vi "FGV_REWORK_login.vi"(6 "login_refnums":T1, 7 "options":T2, 8 "error_in":errorcluster, 9 "access_level_in":i32, 10 "username_in":string, 11 "ID_in":string) -> (0 "error_out":errorcluster, 1 "access_level_out":i32, 2 "username_out":string, 3 "ID_out":string)   [LabVIEW 2019]
uses:
  FGV_REWORK_login.ctl
  REWORK_login_refnums.ctl
  REWORK_destination_selector/FGV_REWORK_destination_selector.ctl
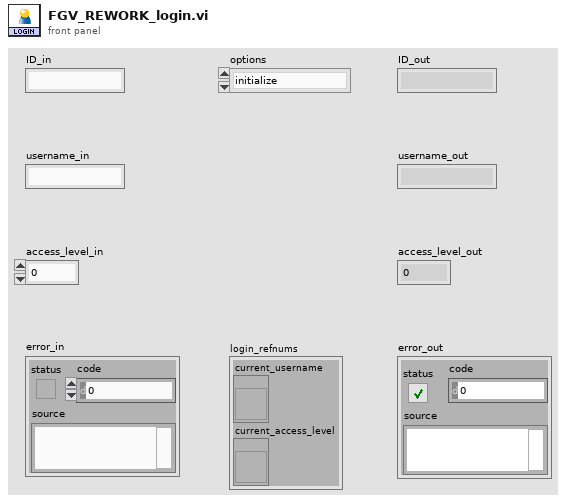
[diagram p1: front panel]
types:
  T1 = typedef "REWORK_login_refnums.ctl" = cluster{"current_username":refnum<vi>, "current_access_level":refnum<vi>}
  T2 = typedef "FGV_REWORK_login.ctl" = enum16{"initialize", "login", "logout", "get_login_info"}
  T3 = typedef "FGV_REWORK_destination_selector.ctl" = enum16{"initialize", "set_values", "display_values", "set_new_login", "enable", "disable", "disable_gray", "get_rework_to", "clear"}
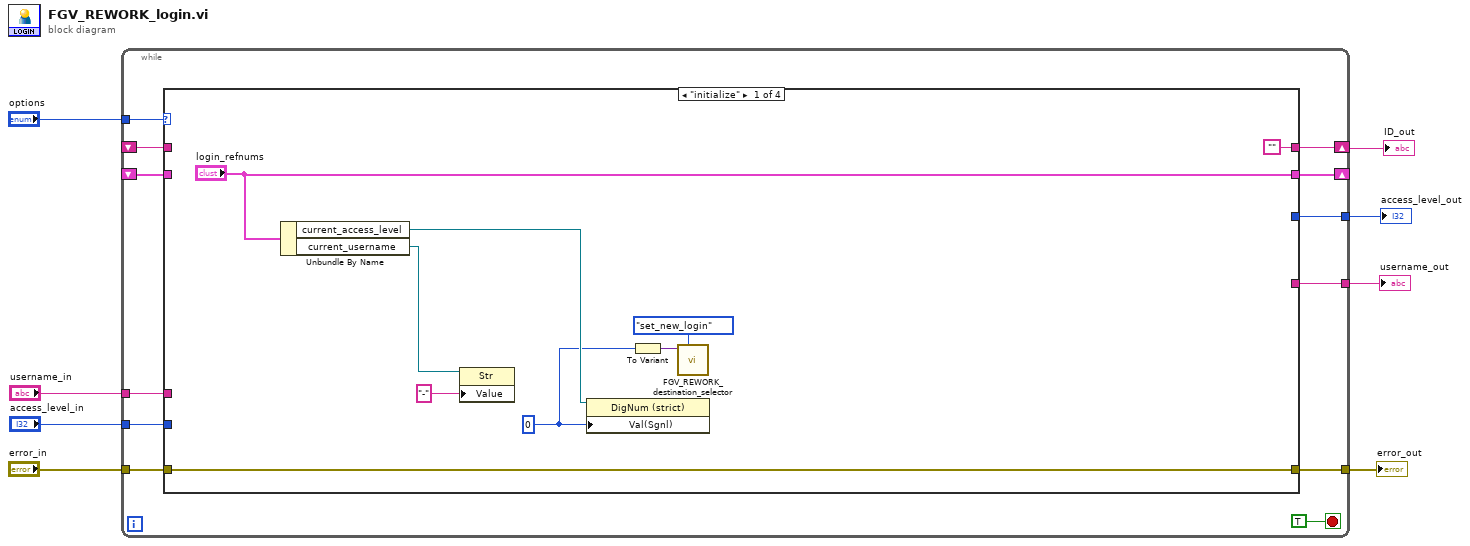
[diagram p0: block diagram]
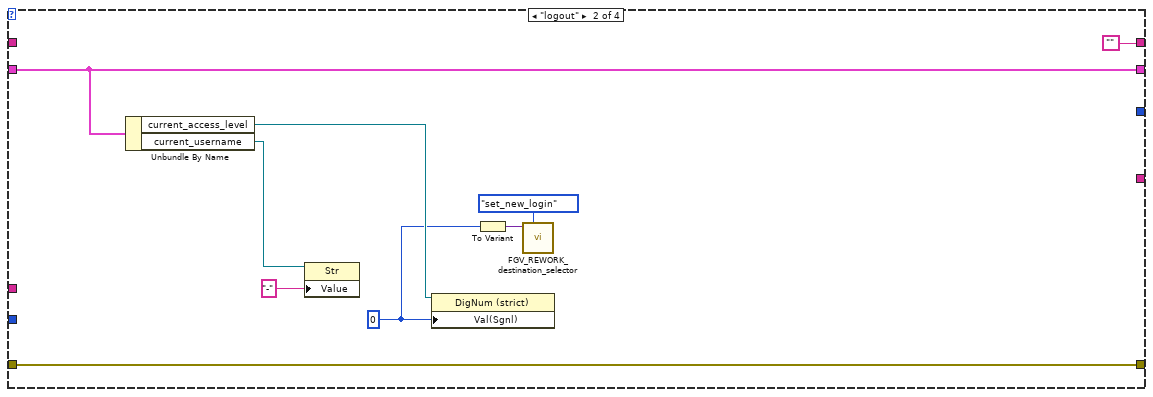
[diagram p2: hidden frame]
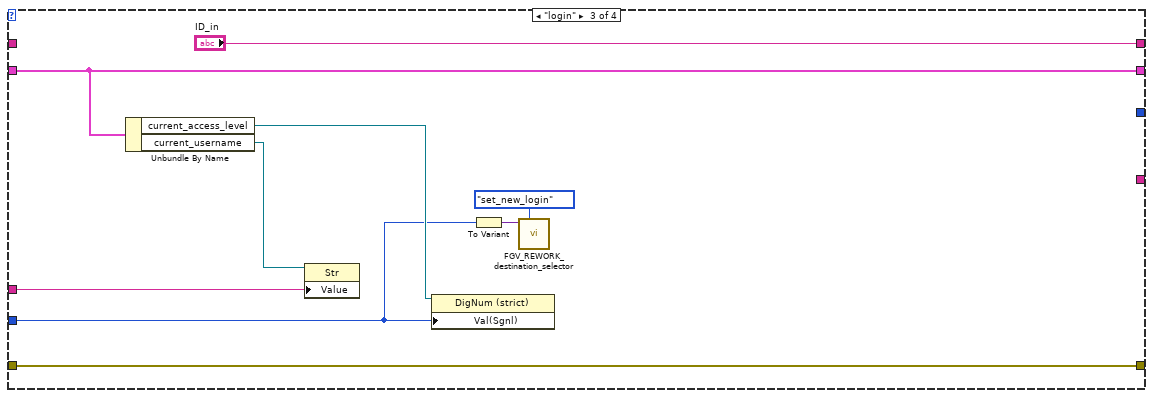
[diagram p3: hidden frame]
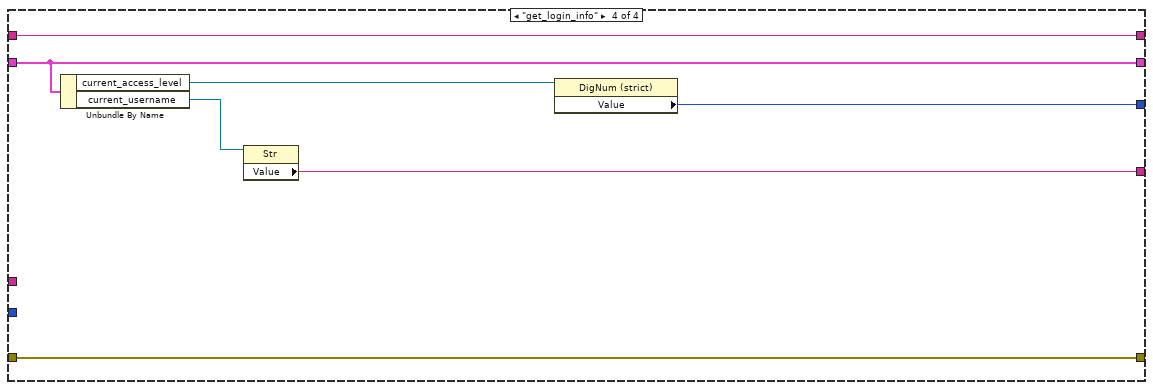
[diagram p4: hidden frame]
diagram:
  n1 = while {
    tunnel: "options" -> [w19]
    tunnel: [w18] -> w8
    tunnel: "error_in" -> [w17]
    shift-right: [w16] -> _
    shift-left: _ -> [w15]
    tunnel: "username_in" -> [w14]
    tunnel: "access_level_in" -> [w13]
    tunnel: [w12] -> w3
    tunnel: [w11] -> w2
    shift-right: [w10] -> w1
    shift-left: _ -> [w9]
    stop <- TRUE stop-if-true
    n2 = case shown="\"initialize\"" w19 {
      tunnel: [w29 w38 w47 w54] -> w18
      tunnel: w17 -> [w29 w38 w47 w54]
      tunnel: ["login_refnums" w34 w43 w53] -> w16
      tunnel: w15 -> [_ w34 w43 w53]
      tunnel: w14 -> [_ _ w46 _]
      tunnel: w13 -> [_ _ w40 _]
      tunnel: [_ _ _ w49] -> w12
      tunnel: [_ _ _ w50] -> w11
      tunnel: ["" "" "ID_in" w48] -> w10
      tunnel: w9 -> [_ _ _ w48]
      frame "initialize" {
        w22 = 0 ("Value")
        n3 = Unbundle By Name("login_refnums") -> ("current_access_level"=w27:refnum<vi>, "current_username"=w28:refnum<vi>)
        n4 = property class="Str"(reference=w28, "Value"="-") -> ()  [unwired: 1 in, 2 out]
        n5 = property class="DigNum (strict)"(reference=w27, "Val(Sgnl)"=w22) -> ()  [unwired: 1 in, 2 out]
        n6 = To Variant(anything=w22) -> (Variant=w23:variant)
        n7 = call "FGV_REWORK_destination_selector.vi"("options"=FGV_REWORK_destination_selector."set_new_login", "input"=w23) -> ()  [unwired: 8 in, 2 out]
      }
      frame "logout" {
        w31 = 0 ("Value")
        n8 = Unbundle By Name(w34) -> ("current_access_level"=w36:refnum<vi>, "current_username"=w37:refnum<vi>)
        n9 = property class="Str"(reference=w37, "Value"="-") -> ()  [unwired: 1 in, 2 out]
        n10 = property class="DigNum (strict)"(reference=w36, "Val(Sgnl)"=w31) -> ()  [unwired: 1 in, 2 out]
        n11 = To Variant(anything=w31) -> (Variant=w32:variant)
        n12 = call "FGV_REWORK_destination_selector.vi"("options"=FGV_REWORK_destination_selector."set_new_login", "input"=w32) -> ()  [unwired: 8 in, 2 out]
      }
      frame "login" {
        n13 = Unbundle By Name(w43) -> ("current_access_level"=w44:refnum<vi>, "current_username"=w45:refnum<vi>)
        n14 = property class="Str"(reference=w45, "Value"=w46) -> ()  [unwired: 1 in, 2 out]
        n15 = property class="DigNum (strict)"(reference=w44, "Val(Sgnl)"=w40) -> ()  [unwired: 1 in, 2 out]
        n16 = To Variant(anything=w40) -> (Variant=w41:variant)
        n17 = call "FGV_REWORK_destination_selector.vi"("options"=FGV_REWORK_destination_selector."set_new_login", "input"=w41) -> ()  [unwired: 8 in, 2 out]
      }
      frame "get_login_info" {
        n18 = Unbundle By Name(w53) -> ("current_access_level"=w51:refnum<vi>, "current_username"=w52:refnum<vi>)
        n19 = property class="Str"(reference=w52) -> ("Value"=w50:string)  [unwired: 1 in, 2 out]
        n20 = property class="DigNum (strict)"(reference=w51) -> ("Value"=w49:i32)  [unwired: 1 in, 2 out]
      }
    }
  }
  "error_out" <- w8
  "access_level_out" <- w3
  "username_out" <- w2
  "ID_out" <- w1
